vi "RunningAverage-RemoveSection.vi"(8 "Error in":errorcluster, 11 "Custom Device ref":T1 format="%.0x") -> (0 "Error out":errorcluster, 3 "Custom Device ref out":T1 format="%.0x")   [LabVIEW 2015, in "Waveform-Processing-Custom-Device Shared.lvlib" / "Running Average.lvlib"]
uses:
  Running Average.lvlib
  <vilib>/NI VeriStand/Custom Device Tools/Custom Device Utility Library/Custom Device Utility Library.lvlib
  <vilib>/NI Veristand/Custom Device Tools/Custom Device Utility Library/NI VeriStand - Search for Item by GUID.vi
  Constants.vi
  Waveform-Processing-Custom-Device Shared.lvlib
  <vilib>/NI VeriStand/Custom Device API/Custom Device API.lvlib
  <vilib>/NI Veristand/Custom Device API/Custom Device Item Ref.ctl
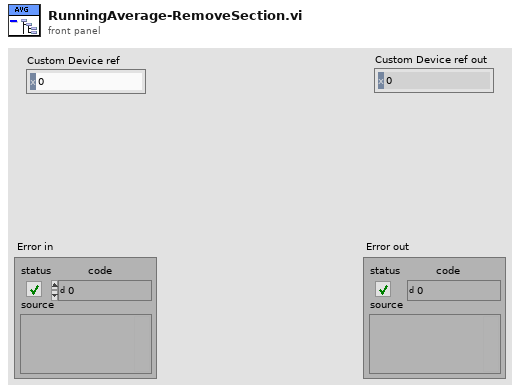
[diagram p1: front panel]
types:
  T1 = typedef "Custom Device API.lvlib/Custom Device Item Ref.ctl" = u64
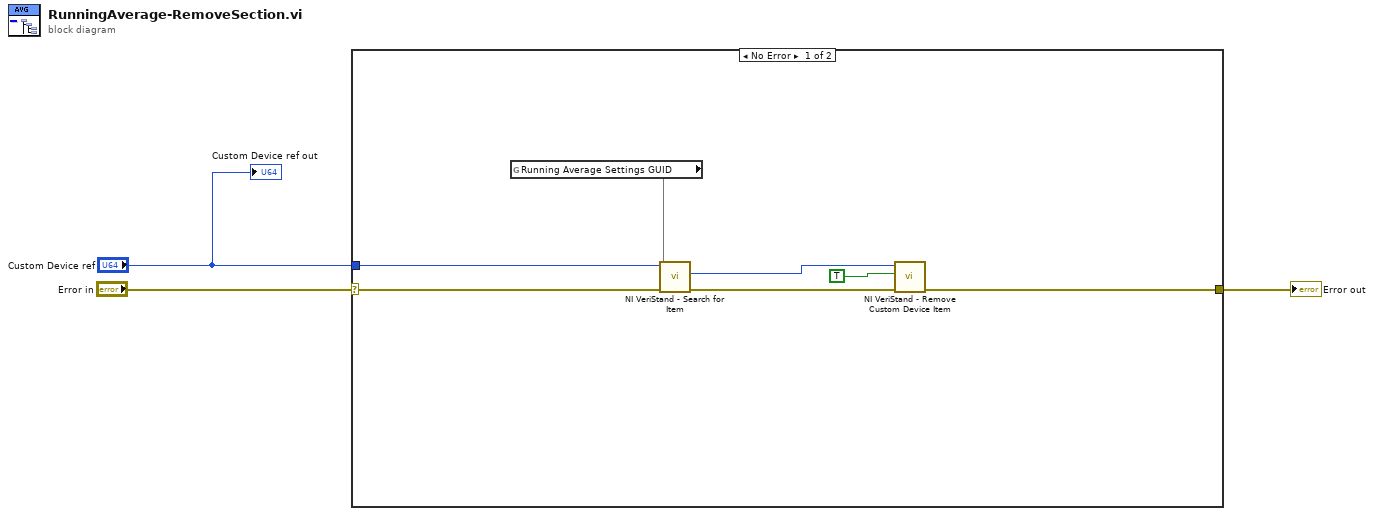
[diagram p0: block diagram]
diagram:
  n1 = case shown="No Error" "Error in" {
    selector: "Error in" -> [w10 w11]
    tunnel: "Custom Device ref" -> [w8 _]
    tunnel: [w5 w11] -> w2
    frame No Error {
      n2 = global read "Constants.vi" "Running Average Settings GUID"() -> (w9)
      n3 = call-poly <vilib>:"NI VeriStand - Search for Item.vi"("error in"=w10, "Item GUID"=w9, "Section Ref in"=w8) -> ("error out"=w7:errorcluster, "Item Ref"=w6:T1)  [unwired: 5 in, 2 out]
      n4 = call <vilib>:"NI VeriStand - Remove Custom Device Item.vi"("error in (no error)"=w7, "Force Delete (F)"=TRUE, "Item Ref in"=w6) -> ("error out"=w5:errorcluster)  [unwired: 7 in, 1 out]
    }
    frame Error {
    }
  }
  "Error out" <- w2
  "Custom Device ref out" <- "Custom Device ref"
